vi "Create Global Command Single Channel_Format.vi"(8 "Error In":errorcluster, 10 "Settings":T1, 11 "Instrument Addon Refnum In":T2=18446744073709551615 format="%.0x") -> (0 "Error Out":errorcluster, 2 "Channel Refnum":T2=18446744073709551615 format="%.0x", 3 "Instrument Addon Refnum Out":T2=18446744073709551615 format="%.0x")   [LabVIEW 2019, in "Scripting API.lvlib"]
uses:
  Scripting API.lvlib
  <vilib>/NI VeriStand/Custom Device API/Custom Device Item Ref.ctl
  Examples/Control 10.ctl
  <vilib>/NI VeriStand/Custom Device API/Custom Device API.lvlib
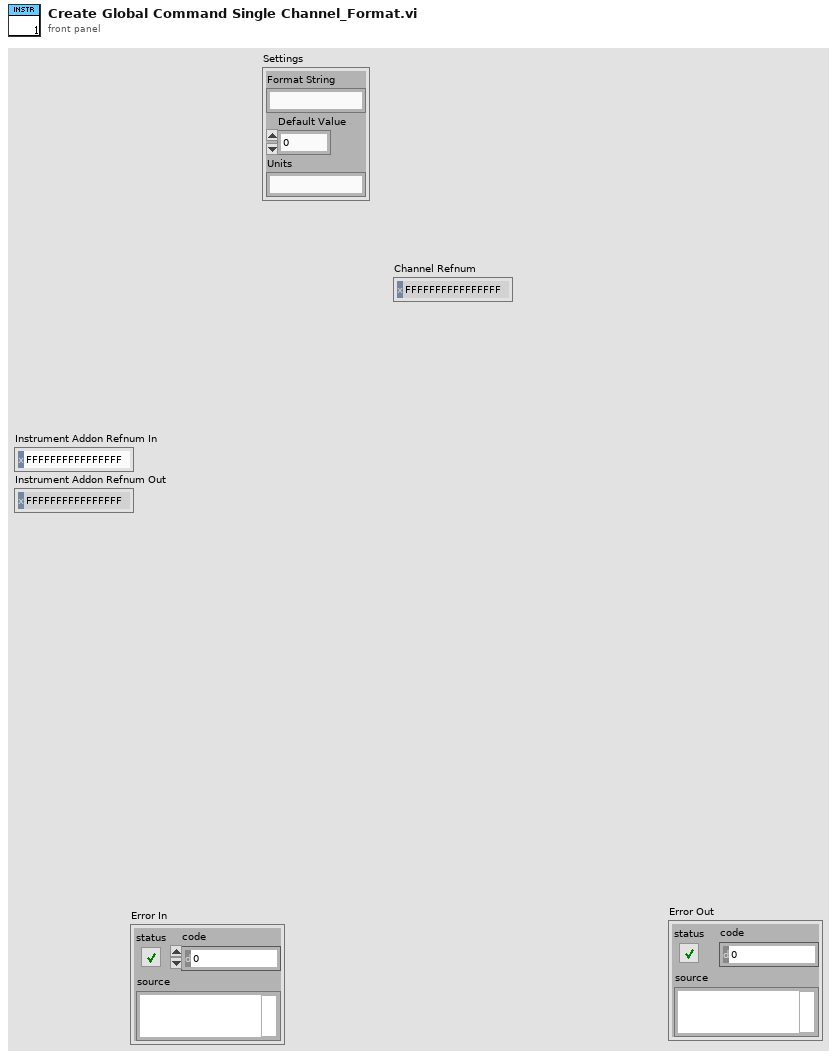
[diagram p1: front panel]
types:
  T1 = typedef "Control 10.ctl" = cluster{"Format String":string, "Default Value":dbl, "Units":string}
  T2 = typedef "Custom Device API.lvlib/Custom Device Item Ref.ctl" = u64
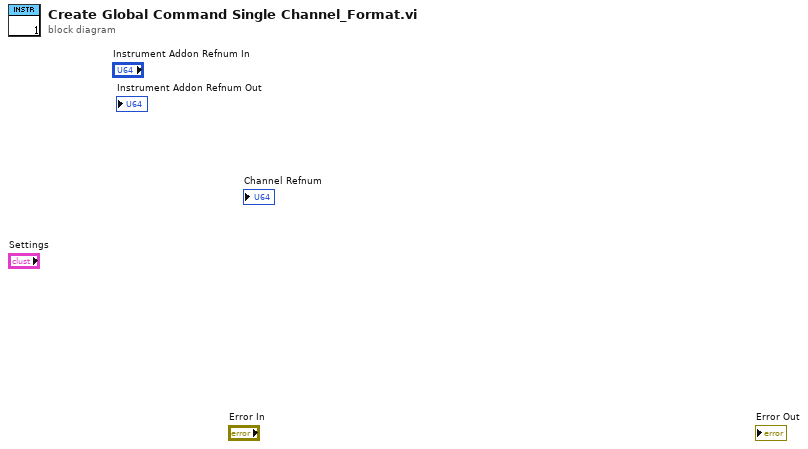
[diagram p0: block diagram]
diagram:
